vi "LEBITVacuum.CryoLevelReading.vi"(4 "error in":errorcluster, 5 "Channels":string, 6 "CRYO VISA resource":refnum<visa-resource-name>) -> (0 "error out":errorcluster, 2 "Data Out":string)   [LabVIEW 2014, in "LEBITVacuum.lvlib"]
uses:
  LEBITVacuum.lvlib
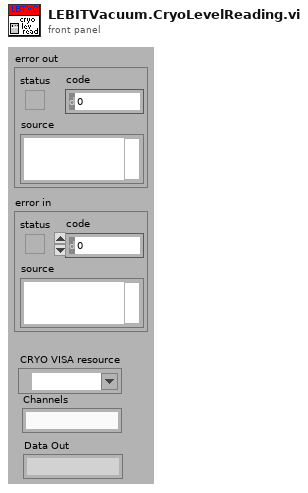
[diagram p1: front panel]
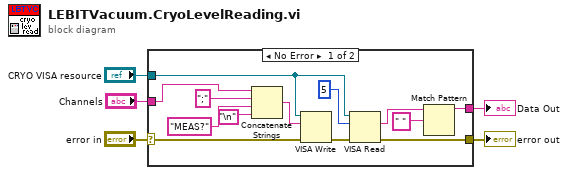
[diagram p0: block diagram]
diagram:
  n1 = case shown="No Error" "error in" {
    selector: "error in" -> [w12 w19]
    tunnel: [w18 w19] -> w5
    tunnel: "Channels" -> [w6 _]
    tunnel: [w14 _] -> w3
    tunnel: "CRYO VISA resource" -> [w13 _]
    frame No Error {
      n2 = Concatenate Strings(w6, ";", "MEAS?" ("data"), "\n") -> (w9:string)
      n3 = VISA Write(VISA resource name=w13, write buffer=w9, error in (no error)=w12) -> (error out=w17:errorcluster)  [unwired: 2 out]
      n4 = VISA Read(VISA resource name=w13, byte count=5, error in (no error)=w17) -> (read buffer=w8:string, error out=w18:errorcluster)  [unwired: 2 out]
      n5 = Match Pattern(string=w8, regular expression=" ") -> (before substring=w14:string)  [unwired: 1 in, 3 out]
    }
    frame Error {
    }
  }
  "error out" <- w5
  "Data Out" <- w3
